vi "PIckPlace tester.vi"() -> ()   [LabVIEW 2017]
uses:
  Shared Components/Gantry Class/Type Definitions/Virtual Modes.ctl
  Shared Components/Gantry Class/Type Definitions/Init_Modes.ctl
  Shared Components/Gantry Class/Gantry Class.lvclass
  Shared Components/Vec3d Class/Vec3d Class.lvclass
panel:
  in  "Virtual Mode":T1=enum."Virtual"
  in  "stop":bool
  out "Image":T2(plugin-control)
  out "error out":errorcluster
  in  "Config Folder":path=path "C:/Users/simra/Desktop/Research/Gantry Purdue/pixel-gantry-control/Config"
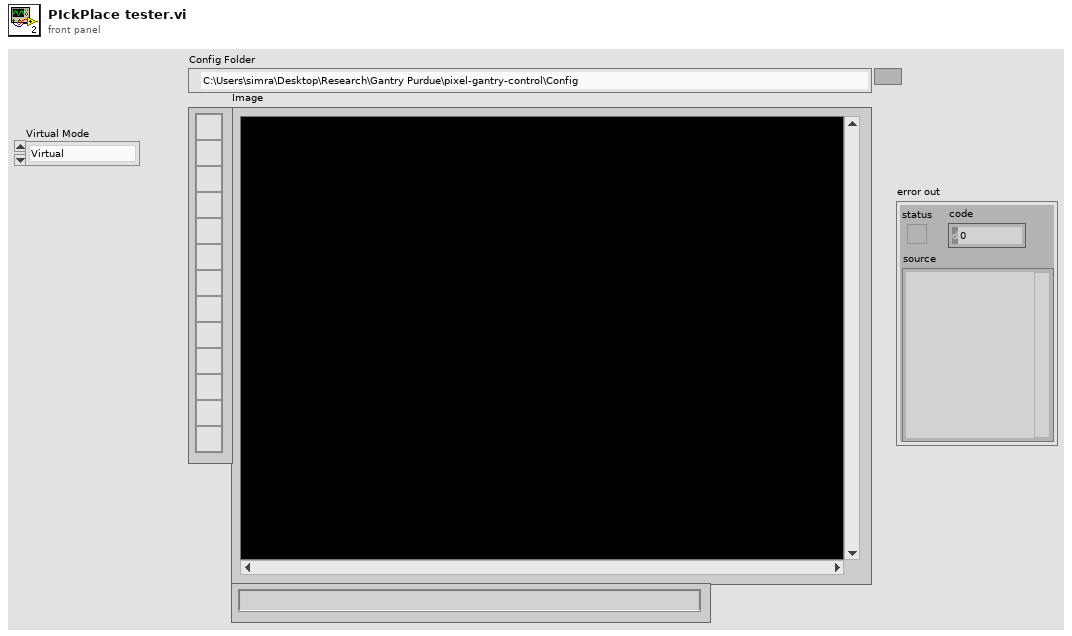
[diagram p1: front panel]
types:
  T1 = typedef "Virtual Modes.ctl" = enum16{"Nonvirtual", "Pseudovirtual", "Virtual"}
  T2 = typedef "IMAQ Image.ctl" = refnum<image>
  T3 = typedef "Init_Modes.ctl" = enum16{"Full", "Robot Only", "Dispenser Only", "Cameras Only", "Robot and Cameras", "Robot and Cameras and Dispenser", "Manifold Only"}
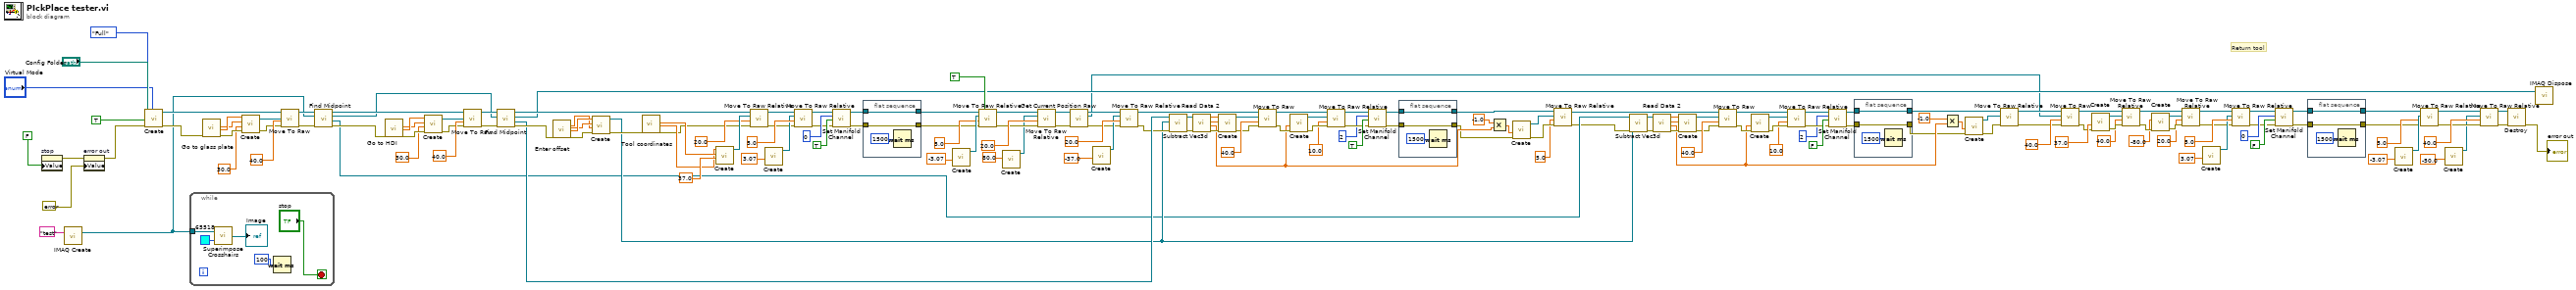
[diagram p0: block diagram]
diagram:
  # "Return tool"
  n1 = property on="stop" class="Bool (strict)"("Value"=FALSE) -> (error out=w172:errorcluster)  [unwired: 2 in, 1 out]
  n2 = call "IMAQ Create"("Image Name"="test") -> ("New Image"=w68:T2)  [unwired: 4 in, 1 out]
  n3 = property on="error out" class="Clust (strict)"(error in=w172, "Value"=errorcluster {"status"=FALSE, "code"=0, "source"=""} ("error in (no error)")) -> (error out=w171:errorcluster)  [unwired: 1 in, 1 out]
  n4 = call "Create.vi"("Virtual Mode"="Virtual Mode", "error in"=w171, "HOME?"=TRUE, "Config Folder"="Config Folder", "Init Mode"=Init_Modes."Full") -> ("error out"=w168:errorcluster, "Gantry out"=w86:refnum<class "Gantry Class.lvclass">)  [unwired: 5 in]
  n5 = while {
    tunnel: w68 -> [w179]
    stop <- "stop" stop-if-true
    n6 = call "Superimpose Crosshairs.vi"("Grid Line Color"=u32 65518, "Refnum in"=w179) -> ("Refnum out"=→"Image":T2)
    n7 = Wait (ms)(milliseconds to wait=u32 100) -> ()  [unwired: 1 out]
  }
  n8 = call "Go to glass plate"("error in (no error)"=w168) -> ("Y"=w166:dbl, "X"=w167:dbl, "error out"=w164:errorcluster)  [unwired: 15 in, 1 out]
  n9 = call "Create.vi"("error in"=w164, "Z"=30.0, "Y"=w166, "X"=w167) -> ("error out"=w85:errorcluster, "Vec3d Class out"=w138:refnum<class "Vec3d Class.lvclass">)  [unwired: 6 in]
  n10 = call-dynamic "Move To Raw.vi"("error in"=w85, "Speed"=40.0, "Destination"=w138, "Gantry in"=w86) -> ("error out"=w77:errorcluster, "Gantry out"=w76:refnum<class "Gantry Class.lvclass">)  [unwired: 6 in]
  n11 = call-dynamic "Find Midpoint.vi"("error in (no error)"=w77, "Image In"=w68, "Gantry Class in"=w76) -> ("error out"=w74:errorcluster, "Vec3d Class out"=w16:refnum<class "Vec3d Class.lvclass">, "Image Out"=w67:T2, "Gantry Class out"=w75:refnum<class "Gantry Class.lvclass">)  [unwired: 5 in]
  n12 = call "Go to HDI"("error in (no error)"=w74) -> ("Y"=w83:dbl, "X"=w84:dbl, "error out"=w81:errorcluster)  [unwired: 15 in, 1 out]
  n13 = call "Create.vi"("error in"=w81, "Z"=30.0, "Y"=w83, "X"=w84) -> ("error out"=w78:errorcluster, "Vec3d Class out"=w80:refnum<class "Vec3d Class.lvclass">)  [unwired: 6 in]
  n14 = call-dynamic "Move To Raw.vi"("error in"=w78, "Speed"=40.0, "Destination"=w80, "Gantry in"=w75) -> ("error out"=w73:errorcluster, "Gantry out"=w72:refnum<class "Gantry Class.lvclass">)  [unwired: 6 in]
  n15 = call-dynamic "Find Midpoint.vi"("error in (no error)"=w73, "Image In"=w67, "Gantry Class in"=w72) -> ("error out"=w70:errorcluster, "Vec3d Class out"=w61:refnum<class "Vec3d Class.lvclass">, "Image Out"=w9:T2, "Gantry Class out"=w71:refnum<class "Gantry Class.lvclass">)  [unwired: 5 in]
  n16 = call "Enter offset"("error in (no error)"=w70) -> ("Z"=w88:dbl, "Y"=w90:dbl, "X"=w91:dbl, "error out"=w89:errorcluster)  [unwired: 14 in, 1 out]
  n17 = call "Create.vi"("error in"=w89, "Z"=w88, "Y"=w90, "X"=w91) -> ("error out"=w64:errorcluster, "Vec3d Class out"=w17:refnum<class "Vec3d Class.lvclass">)  [unwired: 6 in]
  n18 = call "Tool coordinates"("error in (no error)"=w64) -> ("Y"=w66:dbl, "X"=w65:dbl, "error out"=w63:errorcluster)  [unwired: 15 in, 1 out]
  n19 = call "Create.vi"("Z"=37.0, "Y"=w66, "X"=w65) -> ("Vec3d Class out"=w161:refnum<class "Vec3d Class.lvclass">)  [unwired: 7 in, 1 out]
  n20 = call-dynamic "Move To Raw Relative.vi"("error in"=w63, "Speed(mm/s)"=20.0, "Delta"=w161, "Gantry in"=w71) -> ("error out"=w69:errorcluster, "Gantry out"=w153:refnum<class "Gantry Class.lvclass">)  [unwired: 6 in]
  n21 = call "Create.vi"("Z"=3.07) -> ("Vec3d Class out"=w154:refnum<class "Vec3d Class.lvclass">)  [unwired: 9 in, 1 out]
  n22 = call-dynamic "Move To Raw Relative.vi"("error in"=w69, "Speed(mm/s)"=5.0, "Delta"=w154, "Gantry in"=w153) -> ("error out"=w151:errorcluster, "Gantry out"=w152:refnum<class "Gantry Class.lvclass">)  [unwired: 6 in]
  n23 = call-dynamic "Set Manifold Channel.vi"("error in"=w151, "On/Off"=TRUE, "Manifold Channel"=0, "Gantry in"=w152) -> ("error out"=w97:errorcluster, "Gantry out"=w99:refnum<class "Gantry Class.lvclass">)  [unwired: 6 in]
  n24 = flat-sequence {
    tunnel: w99 -> [w184]
    tunnel: [w184] -> w98
    tunnel: w97 -> [w182]
    tunnel: [w182] -> w96
    frame #0 {
      n25 = Wait (ms)(milliseconds to wait=u32 1500) -> ()  [unwired: 1 out]
    }
  }
  n26 = call "Create.vi"("Z"=-3.07) -> ("Vec3d Class out"=w149:refnum<class "Vec3d Class.lvclass">)  [unwired: 9 in, 1 out]
  n27 = call-dynamic "Move To Raw Relative.vi"("Wait?"=TRUE, "error in"=w96, "Speed(mm/s)"=5.0, "Delta"=w149, "Gantry in"=w98) -> ("error out"=w144:errorcluster, "Gantry out"=w145:refnum<class "Gantry Class.lvclass">)  [unwired: 5 in]
  n28 = call "Create.vi"("Y"=80.0 ("Z")) -> ("Vec3d Class out"=w143:refnum<class "Vec3d Class.lvclass">)  [unwired: 9 in, 1 out]
  n29 = call-dynamic "Move To Raw Relative.vi"("error in"=w144, "Speed(mm/s)"=20.0, "Delta"=w143, "Gantry in"=w145) -> ("error out"=w131:errorcluster, "Gantry out"=w133:refnum<class "Gantry Class.lvclass">)  [unwired: 6 in]
  n30 = call-dynamic "Get Current Position Raw.vi"("error in"=w131, "Gantry in"=w133) -> ("error out"=w130:errorcluster, "Vec3d Class out"=w3:refnum<class "Vec3d Class.lvclass">, "Gantry out"=w132:refnum<class "Gantry Class.lvclass">)  [unwired: 7 in]
  n31 = call "Create.vi"("Z"=-37.0) -> ("Vec3d Class out"=w139:refnum<class "Vec3d Class.lvclass">)  [unwired: 9 in, 1 out]
  n32 = call-dynamic "Move To Raw Relative.vi"("error in"=w130, "Speed(mm/s)"=20.0, "Delta"=w139, "Gantry in"=w132) -> ("error out"=w52:errorcluster, "Gantry out"=w50:refnum<class "Gantry Class.lvclass">)  [unwired: 6 in]
  n33 = call "Subtract Vec3d.vi"("error in (no error)"=w52, "Vec3d in 2"=w17, "Vec3d in 1"=w61) -> ("error out"=w54:errorcluster, "Vec3d Class out"=w58:refnum<class "Vec3d Class.lvclass">)  [unwired: 7 in]
  n34 = call-dynamic "Read Data 2.vi"("error in"=w54, "Vec3d in"=w58) -> ("error out"=w53:errorcluster, "Z"=w40:dbl, "Y"=w59:dbl, "X"=w60:dbl)  [unwired: 6 in]
  n35 = call "Create.vi"("error in"=w53, "Y"=w59, "X"=w60) -> ("error out"=w51:errorcluster, "Vec3d Class out"=w57:refnum<class "Vec3d Class.lvclass">)  [unwired: 7 in]
  n36 = call-dynamic "Move To Raw.vi"("error in"=w51, "Speed"=40.0, "Destination"=w57, "Gantry in"=w50) -> ("error out"=w48:errorcluster, "Gantry out"=w56:refnum<class "Gantry Class.lvclass">)  [unwired: 6 in]
  n37 = call "Create.vi"("error in"=w48, "Z"=w40) -> ("error out"=w49:errorcluster, "Vec3d Class out"=w55:refnum<class "Vec3d Class.lvclass">)  [unwired: 8 in]
  n38 = call-dynamic "Move To Raw Relative.vi"("error in"=w49, "Speed(mm/s)"=10.0, "Delta"=w55, "Gantry in"=w56) -> ("error out"=w42:errorcluster, "Gantry out"=w43:refnum<class "Gantry Class.lvclass">)  [unwired: 6 in]
  n39 = call-dynamic "Set Manifold Channel.vi"("error in"=w42, "On/Off"=TRUE, "Manifold Channel"=2, "Gantry in"=w43) -> ("error out"=w44:errorcluster, "Gantry out"=w45:refnum<class "Gantry Class.lvclass">)  [unwired: 6 in]
  n40 = flat-sequence {
    tunnel: w45 -> [w187]
    tunnel: [w187] -> w39
    tunnel: w44 -> [w185]
    tunnel: [w185] -> w38
    frame #0 {
      n41 = Wait (ms)(milliseconds to wait=u32 1500) -> ()  [unwired: 1 out]
    }
  }
  n42 = Multiply(x=-1.0, y=w40) -> (x*y=w136:dbl)
  n43 = call "Create.vi"("error in"=w38, "Z"=w136) -> ("error out"=w134:errorcluster, "Vec3d Class out"=w135:refnum<class "Vec3d Class.lvclass">)  [unwired: 8 in]
  n44 = call-dynamic "Move To Raw Relative.vi"("error in"=w134, "Speed(mm/s)"=5.0, "Delta"=w135, "Gantry in"=w39) -> ("error out"=w10:errorcluster, "Gantry out"=w11:refnum<class "Gantry Class.lvclass">)  [unwired: 6 in]
  n45 = call "Subtract Vec3d.vi"("error in (no error)"=w10, "Vec3d in 2"=w17, "Vec3d in 1"=w16) -> ("error out"=w27:errorcluster, "Vec3d Class out"=w31:refnum<class "Vec3d Class.lvclass">)  [unwired: 7 in]
  n46 = call-dynamic "Read Data 2.vi"("error in"=w27, "Vec3d in"=w31) -> ("error out"=w26:errorcluster, "Z"=w15:dbl, "Y"=w32:dbl, "X"=w33:dbl)  [unwired: 6 in]
  n47 = call "Create.vi"("error in"=w26, "Y"=w32, "X"=w33) -> ("error out"=w25:errorcluster, "Vec3d Class out"=w30:refnum<class "Vec3d Class.lvclass">)  [unwired: 7 in]
  n48 = call-dynamic "Move To Raw.vi"("error in"=w25, "Speed"=40.0, "Destination"=w30, "Gantry in"=w11) -> ("error out"=w23:errorcluster, "Gantry out"=w29:refnum<class "Gantry Class.lvclass">)  [unwired: 6 in]
  n49 = call "Create.vi"("error in"=w23, "Z"=w15) -> ("error out"=w24:errorcluster, "Vec3d Class out"=w28:refnum<class "Vec3d Class.lvclass">)  [unwired: 8 in]
  n50 = call-dynamic "Move To Raw Relative.vi"("error in"=w24, "Speed(mm/s)"=10.0, "Delta"=w28, "Gantry in"=w29) -> ("error out"=w19:errorcluster, "Gantry out"=w20:refnum<class "Gantry Class.lvclass">)  [unwired: 6 in]
  n51 = call-dynamic "Set Manifold Channel.vi"("error in"=w19, "On/Off"=FALSE, "Manifold Channel"=2, "Gantry in"=w20) -> ("error out"=w14:errorcluster, "Gantry out"=w12:refnum<class "Gantry Class.lvclass">)  [unwired: 6 in]
  n52 = flat-sequence {
    tunnel: w12 -> [w190]
    tunnel: [w190] -> w7
    tunnel: w14 -> [w188]
    tunnel: [w188] -> w13
    frame #0 {
      n53 = Wait (ms)(milliseconds to wait=u32 1500) -> ()  [unwired: 1 out]
    }
  }
  n54 = Multiply(x=-1.0, y=w15) -> (x*y=w35:dbl)
  n55 = call "Create.vi"("error in"=w13, "Z"=w35) -> ("error out"=w8:errorcluster, "Vec3d Class out"=w4:refnum<class "Vec3d Class.lvclass">)  [unwired: 8 in]
  n56 = call-dynamic "Move To Raw Relative.vi"("error in"=w8, "Delta"=w4, "Gantry in"=w7) -> ("error out"=w5:errorcluster, "Gantry out"=w6:refnum<class "Gantry Class.lvclass">)  [unwired: 7 in]
  n57 = call-dynamic "Move To Raw.vi"("error in"=w5, "Speed"=40.0, "Destination"=w3, "Gantry in"=w6) -> ("error out"=w125:errorcluster, "Gantry out"=w128:refnum<class "Gantry Class.lvclass">)  [unwired: 6 in]
  n58 = call "Create.vi"("error in"=w125, "Z"=37.0) -> ("error out"=w124:errorcluster, "Vec3d Class out"=w127:refnum<class "Vec3d Class.lvclass">)  [unwired: 8 in]
  n59 = call-dynamic "Move To Raw Relative.vi"("error in"=w124, "Speed(mm/s)"=40.0, "Delta"=w127, "Gantry in"=w128) -> ("error out"=w119:errorcluster, "Gantry out"=w120:refnum<class "Gantry Class.lvclass">)  [unwired: 6 in]
  n60 = call "Create.vi"("error in"=w119, "Y"=-80.0) -> ("error out"=w122:errorcluster, "Vec3d Class out"=w100:refnum<class "Vec3d Class.lvclass">)  [unwired: 8 in]
  n61 = call-dynamic "Move To Raw Relative.vi"("error in"=w122, "Speed(mm/s)"=20.0, "Delta"=w100, "Gantry in"=w120) -> ("error out"=w102:errorcluster, "Gantry out"=w103:refnum<class "Gantry Class.lvclass">)  [unwired: 6 in]
  n62 = call "Create.vi"("Z"=3.07) -> ("Vec3d Class out"=w113:refnum<class "Vec3d Class.lvclass">)  [unwired: 9 in, 1 out]
  n63 = call-dynamic "Move To Raw Relative.vi"("error in"=w102, "Speed(mm/s)"=5.0, "Delta"=w113, "Gantry in"=w103) -> ("error out"=w111:errorcluster, "Gantry out"=w112:refnum<class "Gantry Class.lvclass">)  [unwired: 6 in]
  n64 = call-dynamic "Set Manifold Channel.vi"("error in"=w111, "On/Off"=FALSE, "Manifold Channel"=0, "Gantry in"=w112) -> ("error out"=w93:errorcluster, "Gantry out"=w95:refnum<class "Gantry Class.lvclass">)  [unwired: 6 in]
  n65 = flat-sequence {
    tunnel: w95 -> [w193]
    tunnel: [w193] -> w94
    tunnel: w93 -> [w191]
    tunnel: [w191] -> w92
    frame #0 {
      n66 = Wait (ms)(milliseconds to wait=u32 1500) -> ()  [unwired: 1 out]
    }
  }
  n67 = call "Create.vi"("Z"=-3.07) -> ("Vec3d Class out"=w109:refnum<class "Vec3d Class.lvclass">)  [unwired: 9 in, 1 out]
  n68 = call-dynamic "Move To Raw Relative.vi"("error in"=w92, "Speed(mm/s)"=5.0, "Delta"=w109, "Gantry in"=w94) -> ("error out"=w105:errorcluster, "Gantry out"=w106:refnum<class "Gantry Class.lvclass">)  [unwired: 6 in]
  n69 = call "Create.vi"("Z"=-50.0) -> ("Vec3d Class out"=w104:refnum<class "Vec3d Class.lvclass">)  [unwired: 9 in, 1 out]
  n70 = call-dynamic "Move To Raw Relative.vi"("error in"=w105, "Speed(mm/s)"=40.0, "Delta"=w104, "Gantry in"=w106) -> ("error out"=w2:errorcluster, "Gantry out"=w1:refnum<class "Gantry Class.lvclass">)  [unwired: 6 in]
  n71 = call "Destroy.vi"("error in"=w2, "Gantry Class in"=w1) -> ("error out"=→"error out":errorcluster)  [unwired: 9 in]
  n72 = call "IMAQ Dispose"("Image"=w9) -> ()  [unwired: 5 in, 1 out]
